vi "Install Dependencies.vi"(0 "Export in":refnum<class "Export.lvclass">) -> (4 "Export out":refnum<class "Export.lvclass">)   [LabVIEW 2017, in "CL_G3_VIComponentBuilder.lvlib" / "Export.lvclass"]
doc: "Installs the dependencies required by this export at build time."
uses:
  Export.lvclass
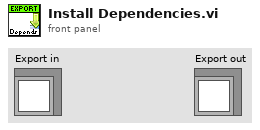
[diagram p1: front panel]
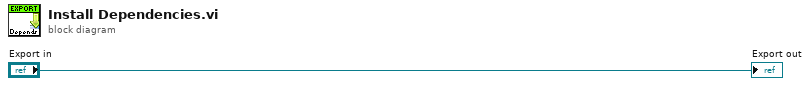
[diagram p0: block diagram]
diagram:
  "Export out" <- "Export in"
